vi "Scenario Update.vi"(8 "error in (no error)":errorcluster, 10 "Scenario (none)":T1, 11 "Connection Refnum":T4) -> (0 "error out":errorcluster, 2 "dup Scenario":T1, 3 "Connection Refnum":T4)   [LabVIEW 2011]
uses:
  Scenario Record.ctl
  Conditions/Condition Record.ctl
  Conditions/Condition Operators.ctl
  Summitek EXT/ODBC/SQL Controls/Connection Refnum.ctl
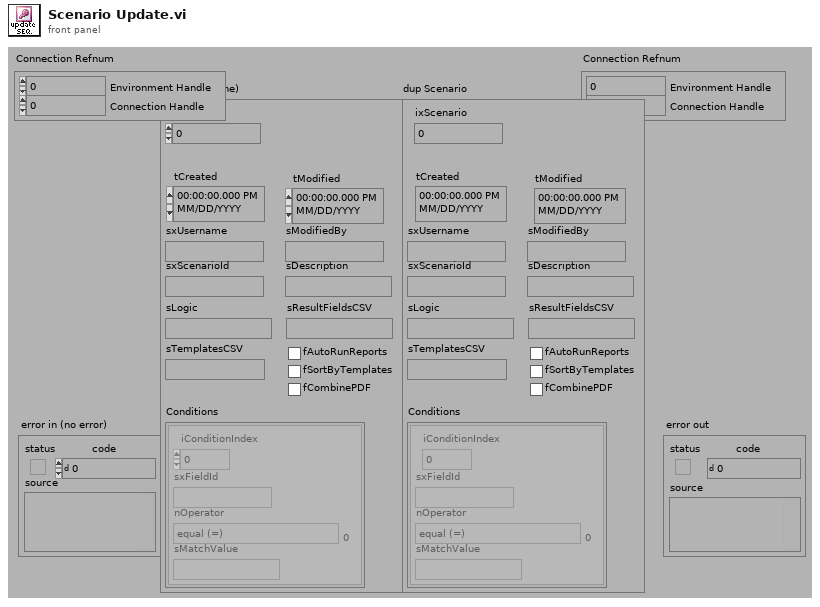
[diagram p1: front panel]
types:
  T1 = typedef "Scenario Record.ctl" = cluster{"ixScenario":i32, "tCreated":timestamp, "tModified":timestamp, "sxUsername":string, "sModifiedBy":string, "sxScenarioId":string, "sDescription":string, "sLogic":string, "sResultFieldsCSV":string, "sTemplatesCSV":string, "fAutoRunReports":bool, "fSortByTemplates":bool, "fCombinePDF":bool, "Conditions":T2[]}
  T2 = typedef "Condition Record.ctl" = cluster{"iConditionIndex":i32, "sxFieldId":string, "nOperator":T3, "sMatchValue":string}
  T3 = typedef "Condition Operators.ctl" = enum16{"equal (=)", "not equal (\\u2260)", "less than (<)", "less than or equal (\\u2264)", "greater than (>)", "greater than or equal (\\u2265)", "contains", "does not contain"}
  T4 = typedef "Connection Refnum.ctl" = cluster{"Environment Handle":i32, "Connection Handle":i32}
  T5 = typedef "Statement Refnum.ctl" = cluster{"Statement Handle":i32, "Parameter Number":u16}
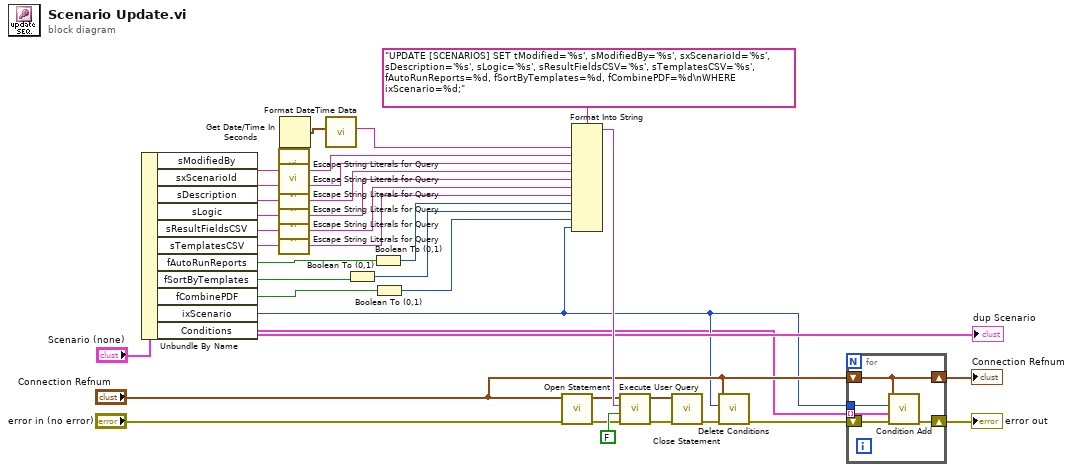
[diagram p0: block diagram]
diagram:
  n1 = Unbundle By Name("Scenario (none)") -> ("sModifiedBy"=w26:string, "sxScenarioId"=w29:string, "sDescription"=w28:string, "sLogic"=w24:string, "sResultFieldsCSV"=w22:string, "sTemplatesCSV"=w9:string, "fAutoRunReports"=w6:bool, "fSortByTemplates"=w2:bool, "fCombinePDF"=w5:bool, "ixScenario"=w14:i32, "Conditions"=w13:T2[])
  n2 = call "Escape String Literals for Query.vi"("String"=w26) -> ("escaped String"=w19:string)  [unwired: 1 in, 13 out]
  n3 = call "Escape String Literals for Query.vi"("String"=w29) -> ("escaped String"=w20:string)  [unwired: 1 in, 13 out]
  n4 = call "Escape String Literals for Query.vi"("String"=w28) -> ("escaped String"=w25:string)  [unwired: 1 in, 13 out]
  n5 = call "Escape String Literals for Query.vi"("String"=w24) -> ("escaped String"=w23:string)  [unwired: 1 in, 13 out]
  n6 = call "Escape String Literals for Query.vi"("String"=w22) -> ("escaped String"=w21:string)  [unwired: 1 in, 13 out]
  n7 = call "Escape String Literals for Query.vi"("String"=w9) -> ("escaped String"=w10:string)  [unwired: 1 in, 13 out]
  n8 = Get Date/Time In Seconds() -> (seconds since 1Jan1904=w7:timestamp)
  n9 = call "Format DateTime Data.vi"("Timestamp in"=w7) -> ("UTC DB String out"=w8:string)  [unwired: 10 out]
  n10 = Boolean To (0,1)(Boolean=w2) -> (0, 1=w1:i16)
  n11 = Boolean To (0,1)(Boolean=w6) -> (0, 1=w4:i16)
  n12 = Boolean To (0,1)(Boolean=w5) -> (0, 1=w3:i16)
  n13 = call "Open Statement.vi"("error in (no error)"="error in (no error)", "Connection Refnum"="Connection Refnum") -> ("error out"=w31:errorcluster, "Statement Refnum"=w30:T5)  [unwired: 4 out]
  n14 = Format Into String(format string="UPDATE [SCENARIOS] SET tModified='%s', sModifiedBy='%s', sxScenarioId='%s', sDescription='%s', sLogic='%s', sResultFieldsCSV='%s', sTemplatesCSV='%s', fAutoRunReports=%d, fSortByTemplates=%d, fCombinePDF=%d\nWHERE ixScenario=%d;" ("User Query"), w8, w19, w20, w25, w23, w21, w10, w4, w1, w3, w14) -> (resulting string=w35:string)  [unwired: 2 in, 1 out]
  n15 = call "Execute User Query.vi"("error in (no error)"=w31, "Return Data? (f)"=FALSE, "User Query"=w35, "Statement Refnum"=w30) -> ("error out"=w32:errorcluster, "Statement Refnum"=w33:T5)  [unwired: 2 out]
  n16 = call "Close Statement.vi"("error in (no error)"=w32, "Statement Refnum"=w33) -> ("error out"=w18:errorcluster)  [unwired: 5 out]
  n17 = call "Delete Conditions.vi"("error in (no error)"=w18, "ixScenario (0)"=w14, "Connection Refnum"="Connection Refnum") -> ("error out"=w12:errorcluster)  [unwired: 1 in, 7 out]
  n18 = for {
    shift-right: [w39] -> w15
    shift-left: "Connection Refnum" -> [w39]
    shift-right: [w40] -> w11
    shift-left: w12 -> [w41]
    tunnel: w13 -> [w38] mode=indexing
    tunnel: w14 -> [w37]
    n19 = call "Condition Add.vi"("error in (no error)"=w41, "Condition"=w38, "ixScenario (0)"=w37, "Connection Refnum"=w39) -> ("error out"=w40:errorcluster)  [unwired: 7 out]
  }
  "error out" <- w11
  "Connection Refnum" <- w15
  "dup Scenario" <- "Scenario (none)"
